vi "UDP.vi"(1 "error in (no error)":errorcluster) -> (0 "error out":errorcluster)   [LabVIEW 2017]
uses:
  Global.vi
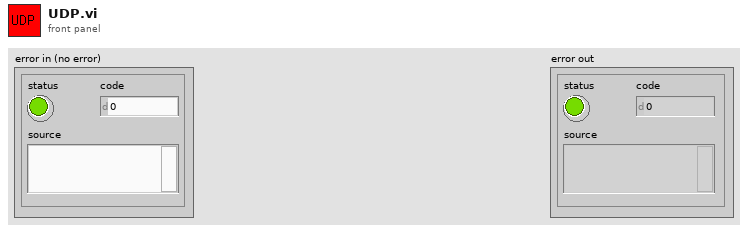
[diagram p1: front panel]
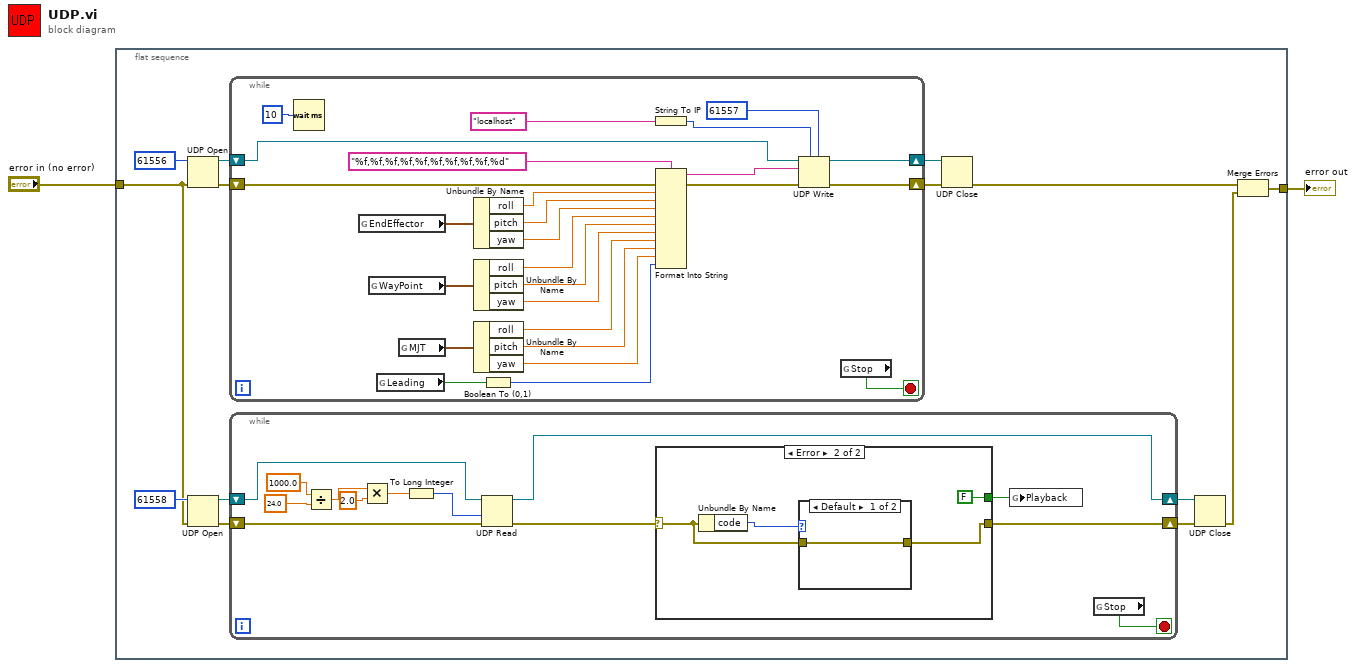
[diagram p0: block diagram]
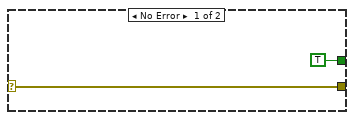
[diagram p2: hidden frame]
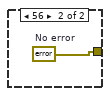
[diagram p3: hidden frame]
diagram:
  n1 = flat-sequence {
    tunnel: "error in (no error)" -> [w8]
    tunnel: [w4] -> w1
    frame #0 {
      n2 = UDP Open(8:w8, 11:u16 61556 ("port")) -> (port=w12:refnum<k16>, 0:w13:errorcluster)  [unwired: 3 in, 1 out]
      n3 = UDP Open(8:w8, 11:u16 61558 ("port")) -> (port=w10:refnum<k16>, 0:w9:errorcluster)  [unwired: 3 in, 1 out]
      n4 = while {
        shift-right: [w63] -> w16
        shift-left: w12 -> [w50]
        shift-right: [w62] -> w15
        shift-left: w13 -> [w49]
        stop <- w57 stop-if-true
        n5 = Wait (ms)(milliseconds to wait=u32 10) -> ()  [unwired: 1 out]
        n6 = global read "Global.vi" "EndEffector"() -> (w51:cluster{"roll":dbl, "pitch":dbl, "yaw":dbl})
        n7 = global read "Global.vi" "WayPoint"() -> (w48:cluster{"roll":dbl, "pitch":dbl, "yaw":dbl})
        n8 = global read "Global.vi" "Leading"() -> (w39:bool)
        n9 = global read "Global.vi" "MJT"() -> (w43:cluster{"roll":dbl, "pitch":dbl, "yaw":dbl})
        n10 = Unbundle By Name(w51) -> ("roll"=w61:dbl, "pitch"=w60:dbl, "yaw"=w59:dbl)
        n11 = Unbundle By Name(w48) -> ("roll"=w47:dbl, "pitch"=w46:dbl, "yaw"=w45:dbl)
        n12 = Unbundle By Name(w43) -> ("roll"=w42:dbl, "pitch"=w41:dbl, "yaw"=w40:dbl)
        n13 = Boolean To (0,1)(Boolean=w39) -> (0, 1=w38:i16)
        n14 = String To IP(1:"localhost" ("name")) -> (0:w54:u32)
        n15 = Format Into String(format string="%f,%f,%f,%f,%f,%f,%f,%f,%f,%d", error in=w49, w61, w60, w59, w47, w46, w45, w42, w41, w40, w38) -> (resulting string=w52:string, error out=w58:errorcluster)  [unwired: 1 in]
        n16 = UDP Write(address=w54, port or service name=u16 61557, connection ID=w50, data in=w52, 8:w58) -> (error out=w62:errorcluster, 3:w63:refnum<k16>)  [unwired: 1 in]
        n17 = global read "Global.vi" "Stop"() -> (w57:bool)
      }
      n18 = while {
        shift-right: [w26] -> w7
        shift-left: w10 -> [w28]
        shift-right: [w17] -> w3
        shift-left: w9 -> [w29]
        stop <- w27 stop-if-true
        n19 = Divide(x=1000.0, y=24.0) -> (x/y=w23:dbl)
        n20 = Multiply(x=w23, y=2.0) -> (x*y=w21:dbl)
        n21 = To Long Integer(number=w21) -> (32bit integer=w20:i32)
        n22 = UDP Read(connection ID=w28, timeout ms (25000)=w20, 8:w29) -> (error out=w19:errorcluster, 3:w26:refnum<k16>)  [unwired: 1 in, 3 out]
        n23 = case shown="Error" w19 {
          selector: w19 -> [w30 w33]
          tunnel: [TRUE ("Playback") FALSE ("Playback")] -> w18
          tunnel: [w30 w34] -> w17
          frame No Error {
          }
          frame Error {
            n24 = Unbundle By Name(w33) -> ("code"=w32:i32)
            n25 = case shown="Default" w32 {
              tunnel: w33 -> [w36 _]
              tunnel: [w36 w37] -> w34
              frame Default {
              }
              frame 56 {
                w37 = errorcluster {"status"=FALSE, "code"=0, "source"=""}  # No error
              }
            }
          }
        }
        n26 = global write "Global.vi" "Playback"(w18) -> ()
        n27 = global read "Global.vi" "Stop"() -> (w27:bool)
      }
      n28 = UDP Close(connection ID=w16, 8:w15) -> (error out=w6:errorcluster)  [unwired: 1 out]
      n29 = UDP Close(connection ID=w7, 8:w3) -> (error out=w5:errorcluster)  [unwired: 1 out]
      n30 = Merge Errors(w6, w5) -> (w4:errorcluster)
    }
  }
  "error out" <- w1
